vi "Write Jobscript for Carbon.vi"(4 "Load VTST for NEB?":bool, 6 "Email?":T2={"Email at Beginning?"=FALSE, "Email at End?"=FALSE, "Email when aborted?"=TRUE}, 8 "Expected Walltime":dbl=172800.0 format="%<%H:%M:%S>t", 9 "Nodes and Processors":T1={"Number of Nodes"=4, "Processors per node"=8}, 10 "CNM Contract Name":string="cnm35383", 11 "Submitname on Carbon":string="Default") -> (3 "Jobscript":string="#!/bin/bash\n\n##  Basics: Number of nodes, processors per node (ppn), and walltime (hhh:mm:ss)\n#PBS -l nodes=4:ppn=8:gen2\n#PBS -l walltime=48:00:00\n#PBS -N derp\n#PBS -A cnm35383 # Robert Klie \n\n## File names for stdout and stderr.  If not set here, the defaults\n## are <JOBNAME>.o<JOBNUM> and <JOBNAME>.e<JOBNUM>\n#PBS -o vasp.out\n#PBS -e err.out\n\n## send mail at begin, end, abort, or never (b, e, a, n)\n#PBS -m a\nmodule unload vasp\nmodule load vasp-vtst\n# change into the directory where qsub will be executed\ncd $PBS_O_WORKDIR\n\n# count allocated cores\nNPROCS=`wc -l < $PBS_NODEFILE`\n\n# start MPI job over default interconnect\nmpirun -machinefile $PBS_NODEFILE -np $NPROCS vasp-vtst\nrm CHG")   [LabVIEW 2010]
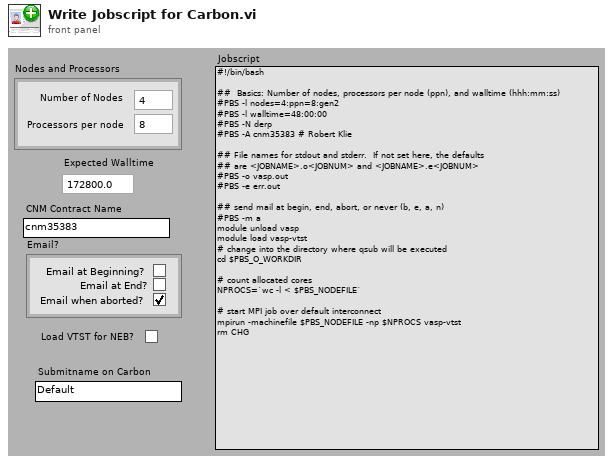
[diagram p1: front panel]
types:
  T1 = cluster{"Number of Nodes":i32, "Processors per node":i32}
  T2 = cluster{"Email at Beginning?":bool, "Email at End?":bool, "Email when aborted?":bool}
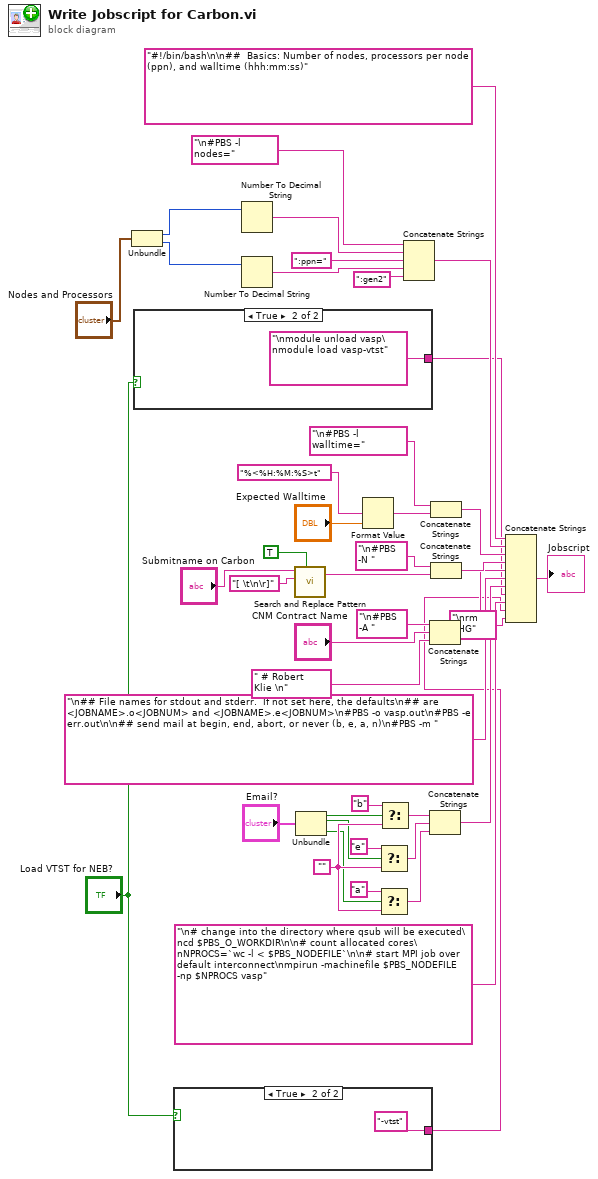
[diagram p0: block diagram]
diagram:
  w40 = ""
  n1 = Unbundle("Nodes and Processors") -> ("Number of Nodes"=w2:i32, "Processors per node"=w1:i32)
  n2 = case shown="True" "Load VTST for NEB?" {
    tunnel: [_ "\nmodule unload vasp\nmodule load vasp-vtst" ("string")] -> w6
    frame False {
    }
    frame True {
    }
  }
  n3 = case shown="True" "Load VTST for NEB?" {
    tunnel: [_ "-vtst" ("string")] -> w4
    frame False {
    }
    frame True {
    }
  }
  n4 = Number To Decimal String(number=w2) -> (decimal integer string=w17:string)  [unwired: 1 in]
  n5 = Number To Decimal String(number=w1) -> (decimal integer string=w15:string)  [unwired: 1 in]
  n6 = call <vilib>:"Search and Replace Pattern.vi"("string"="Submitname on Carbon", "regular expression (\"\")"="[ \t\n\r]" ("regular expression (\"\")"), "replace all? (F)"=TRUE) -> ("result string"=w22:string)  [unwired: 2 in, 1 out]
  n7 = Unbundle("Email?") -> ("Email at Beginning?"=w36:bool, "Email at End?"=w35:bool, "Email when aborted?"=w34:bool)
  n8 = Format Value(format string="%<%H:%M:%S>t", value (0)="Expected Walltime") -> (output string=w26:string)  [unwired: 1 in]
  n9 = Select(t="e", s=w35, f=w40) -> (s? t:f=w38:string)
  n10 = Select(t="a", s=w34, f=w40) -> (s? t:f=w43:string)
  n11 = Select(t="b", s=w36, f=w40) -> (s? t:f=w42:string)
  n12 = Concatenate Strings("\n#PBS -l nodes=", w17, ":ppn=", w15, ":gen2") -> (w12:string)
  n13 = Concatenate Strings("\n#PBS -A " ("string"), "CNM Contract Name", " # Robert Klie \n" ("string")) -> (w7:string)
  n14 = Concatenate Strings(w42, w38, w43) -> (w37:string)
  n15 = Concatenate Strings("\n#PBS -l walltime=", w26) -> (w25:string)
  n16 = Concatenate Strings("\n#PBS -N ", w22) -> (w24:string)
  n17 = Concatenate Strings("#!/bin/bash\n\n##  Basics: Number of nodes, processors per node (ppn), and walltime (hhh:mm:ss)", w12, w25, w24, w7, "\n## File names for stdout and stderr.  If not set here, the defaults\n## are <JOBNAME>.o<JOBNUM> and <JOBNAME>.e<JOBNUM>\n#PBS -o vasp.out\n#PBS -e err.out\n\n## send mail at begin, end, abort, or never (b, e, a, n)\n#PBS -m ", w37, w6, "\n# change into the directory where qsub will be executed\ncd $PBS_O_WORKDIR\n\n# count allocated cores\nNPROCS=`wc -l < $PBS_NODEFILE`\n\n# start MPI job over default interconnect\nmpirun -machinefile $PBS_NODEFILE -np $NPROCS vasp", w4, "\nrm CHG" ("string")) -> (→"Jobscript":string)
